vi "OAT Resample Waveform (Multi Channels).vi"(5 "reset? (True)":bool=TRUE, 6 "max order (auto)":i32, 7 "resolution":u16(ring) items=["normal", "high"], 8 "error in (no error)":errorcluster, 9 "pulse/revolution (1)":i32=1, 10 "speed profile":T2 {"speed [RPM]" format="%.2f"; "time [s]" format="%.2f"}, 11 "scaled signals [EU]":waveform(dbl)[](array[waveform])) -> (0 "error out":errorcluster, 1 "interpolated pulse positions":dbl[](array[numeric]) format="%.2f", 2 "channel info":T1(array[cluster]) {"pregain [dB]" format="%.2f"; "dB reference [EU]" format="%.1e"; "sensor sensitivity [mV/EU]" format="%.2f"}, 3 "resampled signals":cluster{"r0":dbl, "dr":dbl, "Y":dbl[]}[](array[cluster]) {"r0" format="%.2p"; "dr" format="%.2p"; "Y" format="%.2f"})   [LabVIEW 2017]
doc: "Resample the even time sampled <B>scaled signal [EU]</B> to even angle sampled signal."
uses:
  <vilib>/addons/Sound and Vibration/Order Analysis/Tach Process/SubVIs/speed profile.ctl
  <vilib>/addons/Sound and Vibration/Order Analysis/Adv Resampling/oa_Adjust Resample State Info.vi
  <vilib>/addons/Sound and Vibration/Order Analysis/Misc/OAT Error Information.vi
  <vilib>/addons/Sound and Vibration/Order Analysis/Adv Resampling/OAT Prepare Resample Data.vi
  <vilib>/addons/_NISVFA/_Shared subVIs/Common/svc_Engineering Units to Unit Label.vi
  <vilib>/addons/_NISVFA/_Shared subVIs/Common/svc_Unit Label to Engineering Units.vi
  <vilib>/addons/Sound and Vibration/Order Analysis/Resample Order Tracking/SoundVib_Resampling.lvlib
  <vilib>/addons/Sound and Vibration/Order Analysis/Tach Process/SoundVib_TachProcess.lvlib
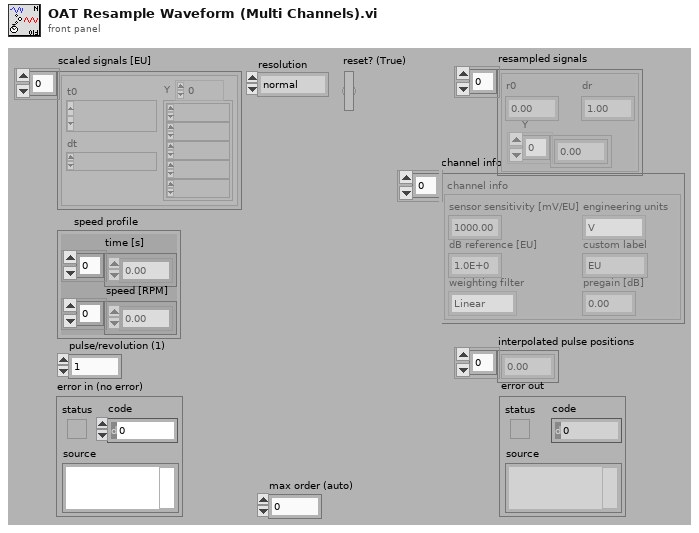
[diagram p1: front panel]
types:
  T1 = cluster{"sensor sensitivity [mV/EU]":dbl, "engineering units":enum16{"custom...", "V", "Pa", "g", "m/s^2", "m/s", "m", "in/s^2", "in/s", "in"}, "dB reference [EU]":dbl, "custom label":string, "weighting filter":enum16{"Linear", "A-weighting", "B-weighting", "C-weighting"}, "pregain [dB]":dbl}[]
  T2 = typedef "SoundVib_TachProcess.lvlib/speed profile.ctl" = cluster{"time [s]":dbl[], "speed [RPM]":dbl[]}
  T3 = typedef "svc_Channel Info.ctl" = cluster{"sensor sensitivity":dbl, "engineering units":T4, "dB reference":dbl, "custom label":string, "weighting filter":T5, "pregain":dbl}
  T4 = typedef "svc_Engineering Units Text Ring.ctl" = u16
  T5 = typedef "svc_Weighting Filter Text Ring.ctl" = u16
  T6 = typedef "OAT Resample Filter Prototype.ctl" = cluster{"left wing":dbl[], "increment":dbl[], "max dec":i32, "timing jitter":enum32{"Interpolation", "Rounding"}, "band limiting?":bool}
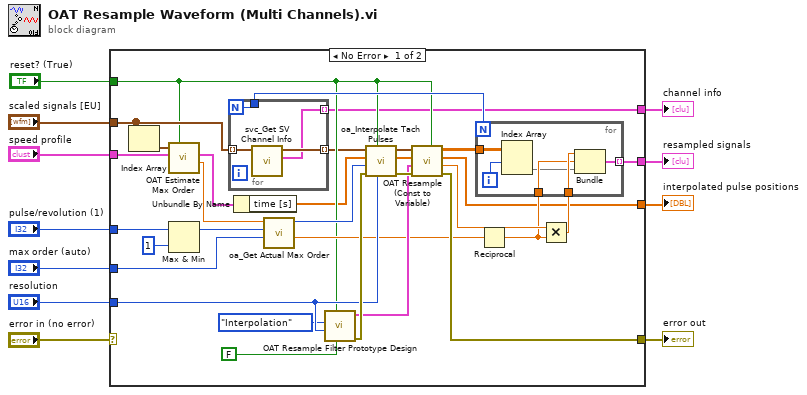
[diagram p0: block diagram]
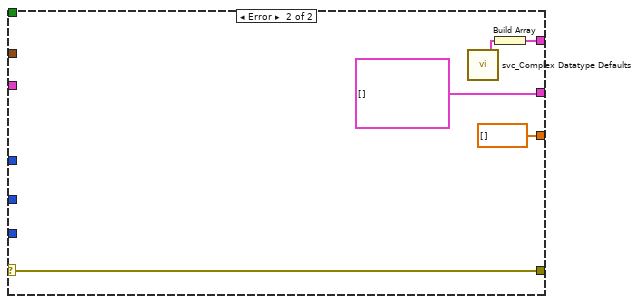
[diagram p2: hidden frame]
diagram:
  n1 = case shown="No Error" "error in (no error)" {
    selector: "error in (no error)" -> [_ w57]
    tunnel: "pulse/revolution (1)" -> [w42 _]
    tunnel: "max order (auto)" -> [w23 _]
    tunnel: [w41 cluster{dbl, dbl, "Y":dbl[]}[] []] -> w3
    tunnel: "scaled signals [EU]" -> [w28 _]
    tunnel: "speed profile" -> [w36 _]
    tunnel: [w34 dbl[] [] ("time stamps")] -> w8
    tunnel: "reset? (True)" -> [w18 _]
    tunnel: [w33 w57] -> w6
    tunnel: "resolution" -> [w21 _]
    tunnel: [w17 w54] -> w1
    frame No Error {
      n2 = Index Array(array=w28) -> (element=w27:waveform(dbl))  [unwired: 1 in]
      n3 = call <vilib>:"OAT Estimate Max Order.vi"("reset? (True)"=w18, "speed profile in"=w36, "scaled signal [EU] in"=w27) -> ("max suggested order"=w24:dbl, "speed profile out"=w35:T2)  [unwired: 5 in, 2 out]
      n4 = Max & Min(x=w42, y=1) -> (max(x,y)=w20:i32)  [unwired: 1 out]
      n5 = for {
        N -> [w50]
        tunnel: w28 -> [w52] mode=indexing
        tunnel: [w51] -> w14 mode=indexing
        tunnel: [w50] -> w25
        tunnel: [w49] -> w17 mode=indexing
        n6 = call <vilib>:"svc_Get SV Channel Info.vi"("scaled signal [EU]"=w52) -> ("channel info"=w49:T3, "dup scaled signal [EU]"=w51:waveform(dbl))  [unwired: 5 in, 4 out]
      }
      n7 = Unbundle By Name(w35) -> ("time [s]"=w12:dbl[])
      n8 = call <vilib>:"oa_Get Actual Max Order.vi"("max order (auto)"=w23, "pulse/revolution (1)"=w20, "max suggested order"=w24) -> ("new pulse/revolution"=w19:dbl, "interpolation factor"=w22:i32)  [unwired: 7 in]
      n9 = call <vilib>:"OAT Resample Filter Prototype Design.vi"("alias free"=FALSE ("alias protect in final transition"), "reset? (True)"=w18, "resolution"=w21, "timing jitter"=enum32{"Interpolation", "Rounding"}."Interpolation") -> ("error out"=w32:errorcluster, "filter prototype"=w29:T6)  [unwired: 5 in, 1 out]
      n10 = call <vilib>:"oa_Interpolate Tach Pulses.vi"("resolution"=w21, "reset? (True)"=w18, "error in (no error)"=w32, "interpolation factor"=w22, "pulse positions [s]"=w12, "scaled signals (EU)"=w14) -> ("error out"=w31:errorcluster, "interpolated pulse positions[s]"=w13:dbl[], "dup scaled signals (EU)"=w15:waveform(dbl)[])  [unwired: 2 in, 1 out]
      n11 = call <vilib>:"OAT Resample (Const to Variable).vi"("reset? (True)"=w18, "error in (no error)"=w31, "filter prototype"=w29, "time"=w13, "scaled signals (EU)"=w15) -> ("error out"=w33:errorcluster, "offset"=w38:dbl, "time stamps"=w34:dbl[], "Y"=w26:dbl[][])  [unwired: 3 in]
      n12 = Reciprocal(x=w19) -> (1/x=w37:dbl)
      n13 = Multiply(x=w38, y=w37) -> (x*y=w39:dbl)
      n14 = for {
        N: w25 -> [_]
        tunnel: [w48] -> w41 mode=indexing
        tunnel: w39 -> [w47]
        tunnel: w37 -> [w46]
        tunnel: w26 -> [w45]
        i -> [w44]
        n15 = Index Array(array=w45, index (row)=w44) -> (element=w43:dbl[])  [unwired: 1 in]
        n16 = Bundle(w47, w46, "Y"=w43) -> (w48:cluster{dbl, dbl, "Y":dbl[]})  [unwired: 1 in]
      }
    }
    frame Error {
      n17 = call <vilib>:"svc_Complex Datatype Defaults.vi"() -> ("channel info"=w53:T3)  [unwired: 11 in, 8 out]
      n18 = Build Array(w53) -> (w54:T3[])
    }
  }
  "interpolated pulse positions" <- w8
  "error out" <- w6
  "resampled signals" <- w3
  "channel info" <- w1
